vi "BarcodeprintR92B.vi"() -> ()   [LabVIEW 2020]
panel:
  out "error out":errorcluster
  in  "错误输入（无错误）":errorcluster
  in  "单选按钮":enum32{"保存", "打印"}(radio)=enum."打印"
  out "二维码图片":picture
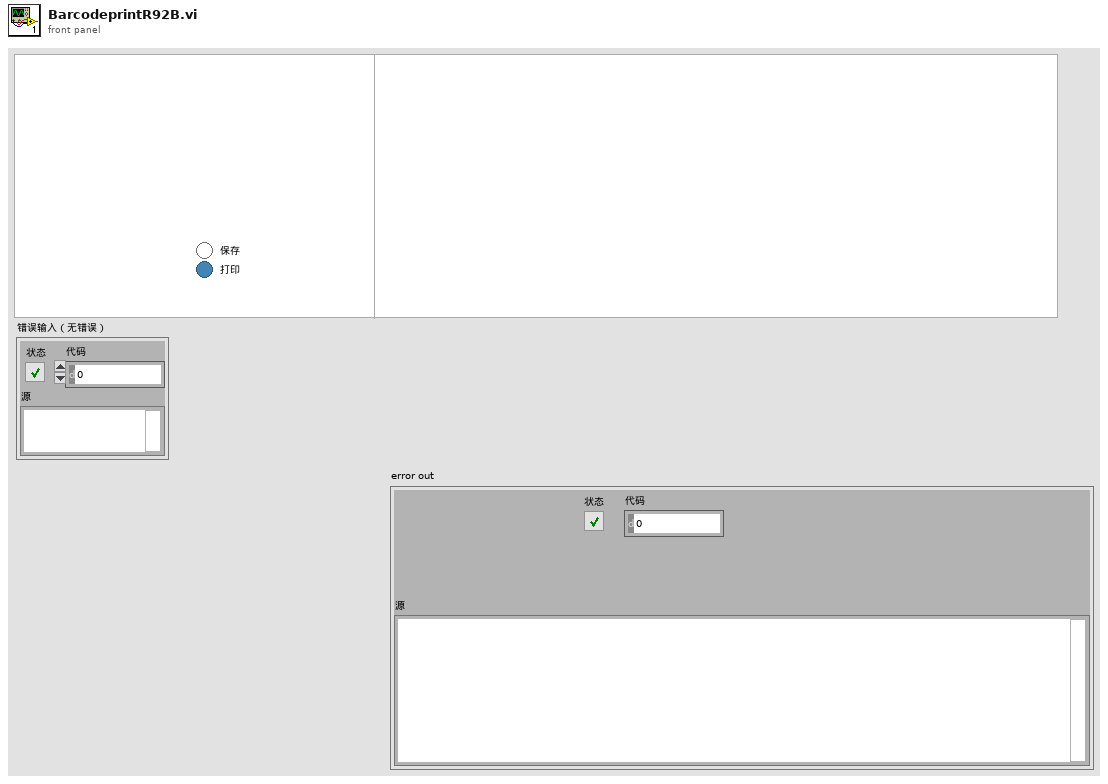
[diagram p1: front panel]
types:
  T1 = typedef "imagedata.ctl" = cluster{"image type":i32, "image depth":i32, "image":u8[], "mask":u8[], "colors":u32[], "Rectangle":cluster{"left":i16, "top":i16, "right":i16, "bottom":i16}}
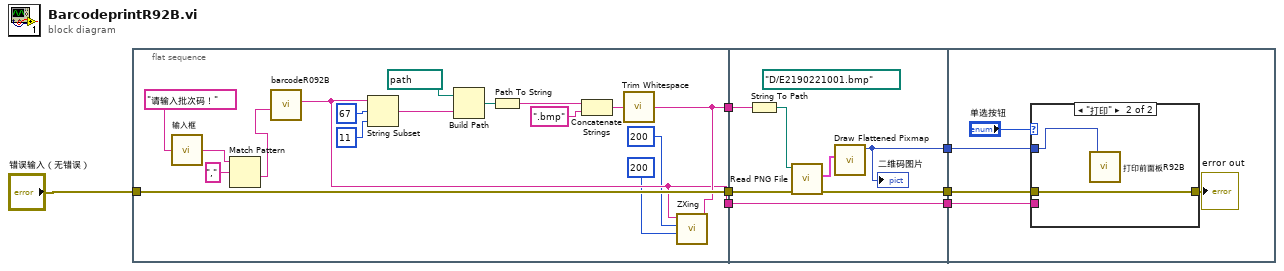
[diagram p0: block diagram]
diagram:
  n1 = flat-sequence {
    tunnel: "错误输入（无错误）" -> [w24]
    tunnel: [w24] -> w5
    tunnel: [w14] -> w4
    tunnel: [w15] -> w1
    tunnel: w5 -> [w31]
    tunnel: [w29] -> w7
    tunnel: w4 -> [w28]
    tunnel: [w28] -> w3
    tunnel: [w27] -> w2
    tunnel: w1 -> [w26]
    tunnel: w7 -> [w35]
    tunnel: w3 -> [w33]
    tunnel: w2 -> [w32]
    frame #0 {
      n2 = call "输入框.vi"("提示信息"="请输入批次码！") -> ("条形码输出"=w9:string)
      n3 = Match Pattern(string=w9, regular expression="," ("正则表达式")) -> (after substring=w8:string)  [unwired: 1 in, 3 out]
      n4 = call "barcodeR092B.vi"("主码"=w8) -> ("R92A二维码"=w14:string)  [unwired: 9 in]
      n5 = String Subset(string=w14, offset (0)=67 ("偏移量(0)"), length (rest)=11 ("长度（剩余）")) -> (substring=w16:string)
      n6 = Build Path(base path=path "D:/条码" ("基路径"), name or relative path=w16) -> (appended path=w21:path)
      n7 = Path To String(path=w21) -> (string=w19:string)
      n8 = Concatenate Strings(w19, ".bmp" ("字符串")) -> (w20:string)
      n9 = call <vilib>:"Trim Whitespace.vi"("string"=w20) -> ("trimmed string"=w15:string)  [unwired: 1 in]
      n10 = call "ZXing.vi"("二维码保存路径"=w15, "height"=200, "width"=200, "contents"=w14) -> ()  [unwired: 7 in, 1 out]
    }
    frame #1 {
      (unwired) path "D:/E2190221001.bmp" ("path to BMP file")
      n11 = String To Path(string=w26) -> (path=w25:path)
      n12 = call <vilib>:"Read PNG File.vi"("error in (no error)"=w31, "path to PNG file"=w25) -> ("error out"=w29:errorcluster, "image data"=w30:T1)  [unwired: 7 in, 1 out]
      n13 = call <vilib>:"Draw Flattened Pixmap.vi"("image data"=w30) -> ("new picture"=w27:picture)  [unwired: 8 in]
      "二维码图片" <- w27
    }
    frame #2 {
      n14 = case shown="\"打印\"" "单选按钮" {
        tunnel: w35 -> [w37 w39]
        tunnel: [w37 w39] -> w34
        tunnel: w33 -> [_ _]
        tunnel: w32 -> [_ w38]
        frame "保存", Default {
        }
        frame "打印" {
          n15 = call "打印前面板R92B.vi"("二维图片 2"=w38) -> ()  [unwired: 8 in]
        }
      }
      "error out" <- w34
    }
  }
